vi "chgCfgDir2.vi"(10 "Path":path=path "C:/Etion Projects/HTSTE2/StationGlobals edit - Copy", 11 "Application Manager":refnum<k7>(container)) -> (0 "error out":errorcluster)   [LabVIEW 2015]
panel:
  in  "error in (no error)":errorcluster
  # "C:\\Etion Projects\\HTSTE2\\StationGlobals edit - Copy"
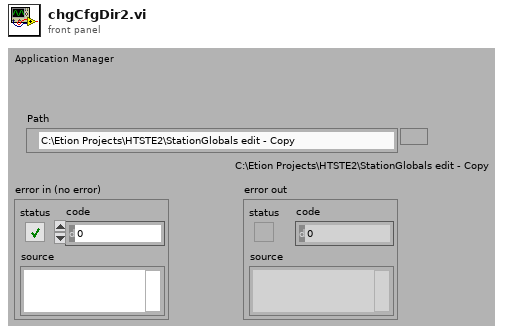
[diagram p1: front panel]
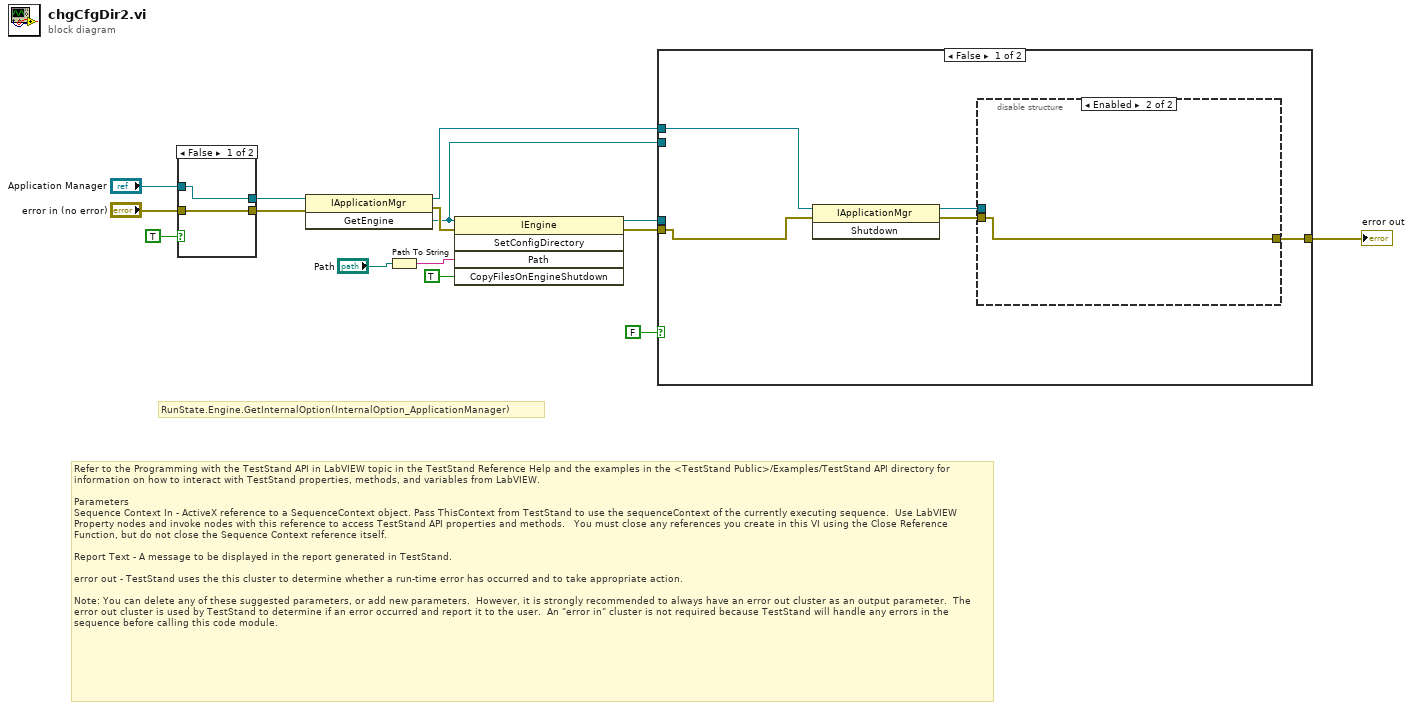
[diagram p0: block diagram]
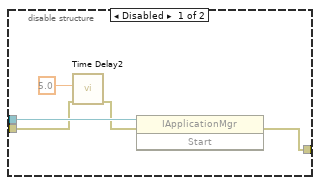
[diagram p2: hidden frame]
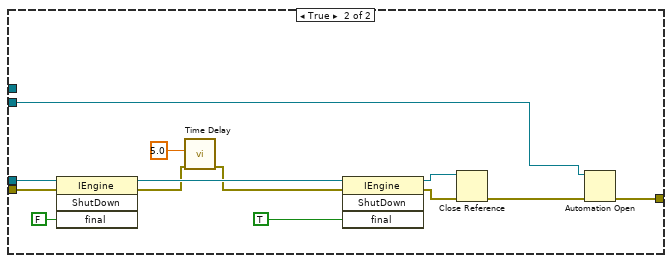
[diagram p3: hidden frame]
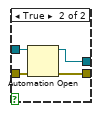
[diagram p4: hidden frame]
diagram:
  # "RunState.Engine.GetInternalOption(InternalOption_ApplicationManager)"
  # "Refer to the Programming with the TestStand API in LabVIEW topic in the TestStand Reference Help and the examples in the <TestStand Public>/Examples/TestStand API directory for information on how to interact with TestStand properties, methods, and variables from LabVIEW.\n\nParameters\nSequence Context In - ActiveX reference to a SequenceContext object. Pass ThisContext from TestStand to use the sequenceContext of the currently executing sequence.  Use LabVIEW Property nodes and invoke nodes with this reference to access TestStand API properties and methods.   You must close any references you create in this VI using the Close Reference Function, but do not close the Sequence Context reference itself.\n\nReport Text - A message to be displayed in the report generated in TestStand. \n\nerror out - TestStand uses the this cluster to determine whether a run-time error has occurred and to take appropriate action.  \n\nNote: You can delete any of these suggested parameters, or add new parameters.  However, it is strongly recommended to always have an error out cluster as an output parameter.  The error out cluster is used by TestStand to determine if an error occurred and report it to the user.  An \"error in\" cluster is not required because TestStand will handle any errors in the sequence before calling this code module."
  n1 = case shown="False" TRUE {
    tunnel: "Application Manager" -> [w16 w21]
    tunnel: "error in (no error)" -> [w17 w20]
    tunnel: [w17 w19] -> w13
    tunnel: [w16 w18] -> w12
    frame False {
    }
    frame True {
      n2 = Automation Open(error in (no error)=w20, Automation Refnum=w21) -> (Automation Refnum=w18:refnum<k7>, error out=w19:errorcluster)  [unwired: 2 in]
    }
  }
  n3 = invoke class="IApplicationMgr" method="GetEngine"(reference=w12, error in=w13) -> (reference out=w1:refnum<k7>, error out=w9:errorcluster, "GetEngine"=w3:refnum<k7>)  [unwired: 1 in]
  n4 = Path To String(path="Path") -> (string=w8:string)
  n5 = invoke class="IEngine" method="SetConfigDirectory"(reference=w3, error in=w9, "Path"=w8, "CopyFilesOnEngineShutdown"=TRUE) -> (reference out=w11:refnum<k7>, error out=w10:errorcluster)  [unwired: 1 in, 3 out]
  n6 = case shown="False" FALSE {
    tunnel: w11 -> [_ w45]
    tunnel: w10 -> [w26 w44]
    tunnel: [w23 w34] -> w4
    tunnel: w3 -> [_ w33]
    tunnel: w1 -> [w25 _]
    frame False {
      n7 = invoke class="IApplicationMgr" method="Shutdown"(reference=w25, error in=w26) -> (reference out=w24:refnum<k7>, error out=w22:errorcluster)  [unwired: 1 in, 1 out]
      n8 = disable-structure shown="Enabled" {
        disable-tunnel: w24 -> [w31 _]
        disable-tunnel: [w30 w32] -> w23
        disable-tunnel: w22 -> [w28 w32]
        frame Disabled {
          n9 = call "Time Delay2"("error in (no error)"=w28, "Delay Time (s)"=5.0) -> ("error out"=w27:errorcluster)  [unwired: 9 in]
          n10 = invoke class="IApplicationMgr" method="Start"(reference=w31, error in=w27) -> (error out=w30:errorcluster)  [unwired: 1 in, 2 out]
        }
        frame Enabled {
        }
      }
    }
    frame True {
      n11 = invoke class="IEngine" method="ShutDown"(reference=w45, error in=w44, "final"=FALSE) -> (reference out=w41:refnum<k7>, error out=w38:errorcluster)  [unwired: 1 in, 2 out]
      n12 = call "Time Delay"("error in (no error)"=w38, "Delay Time (s)"=5.0) -> ("error out"=w37:errorcluster)  [unwired: 9 in]
      n13 = invoke class="IEngine" method="ShutDown"(reference=w41, error in=w37, "final"=TRUE) -> (reference out=w39:refnum<k7>, error out=w40:errorcluster)  [unwired: 1 in, 2 out]
      n14 = Close Reference(reference=w39, error in (no error)=w40) -> (error out=w35:errorcluster)
      n15 = Automation Open(error in (no error)=w35, Automation Refnum=w33) -> (error out=w34:errorcluster)  [unwired: 2 in, 1 out]
    }
  }
  "error out" <- w4
